vi "LithographyDriver.vi"(8 "error in (no error)":errorcluster) -> (0 "error out":errorcluster)   [LabVIEW 2016]
uses:
  Controls/lithography_Control.ctl
  litho folder/Global/Lithography Data.vi
  Desktop/Signal IO/SignalIO/tipvoltageglobal.vi
panel:
  in  "References":T1
  out "Current Object:":string
  out "Status:":string
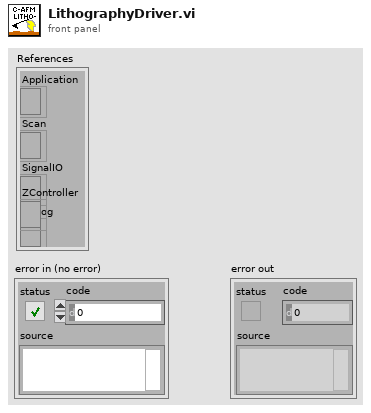
[diagram p1: front panel]
types:
  T1 = cluster{"Scan":refnum<k7>, "Lithog":refnum<k7>, "Application":refnum<k7>, "SignalIO":refnum<k7>, "ZController":refnum<k7>}
  T2 = typedef "lithography_Control.ctl" = enum16{"open_app", "create_ref", "current_pos", "init_litho", "get_init_pt", "clear_litho", "set_param", "move_tip", "create_queue", "clean_up_litho", "start_litho", "end"}
  T3 = cluster{"X_offset":dbl, "Y_offset":dbl, "init_x":dbl, "init_y":dbl, "voltage":dbl}
  T4 = cluster{"Name":string, "Litho":cluster{"X":dbl, "Y":dbl, "Speed":dbl, "Voltage":dbl}[]}[]
  T5 = cluster{"Lithography Data Out":cluster{"Name":string, "Litho":cluster{"X":dbl, "Y":dbl, "Speed":dbl, "Voltage":dbl}[]}[], "Values":cluster{"X_offset":dbl, "Y_offset":dbl, "init_x":dbl, "init_y":dbl, "voltage":dbl}, "References":cluster{"Scan":refnum<k7>, "Lithog":refnum<k7>, "Application":refnum<k7>, "SignalIO":refnum<k7>, "ZController":refnum<k7>}}
  T6 = cluster{"Pattern Data":cluster{"Name":string, "Litho":cluster{"X":dbl, "Y":dbl, "Speed":dbl, "Voltage":dbl}[]}, "Values":cluster{"X_offset":dbl, "Y_offset":dbl, "init_x":dbl, "init_y":dbl, "voltage":dbl}, "References":cluster{"Scan":refnum<k7>, "Lithog":refnum<k7>, "Application":refnum<k7>, "SignalIO":refnum<k7>, "ZController":refnum<k7>}}
  T7 = cluster{"X":dbl, "Y":dbl, "Speed":dbl, "Voltage":dbl}[]
  T8 = cluster{"X":dbl, "Y":dbl, "Speed":dbl, "Voltage":dbl}
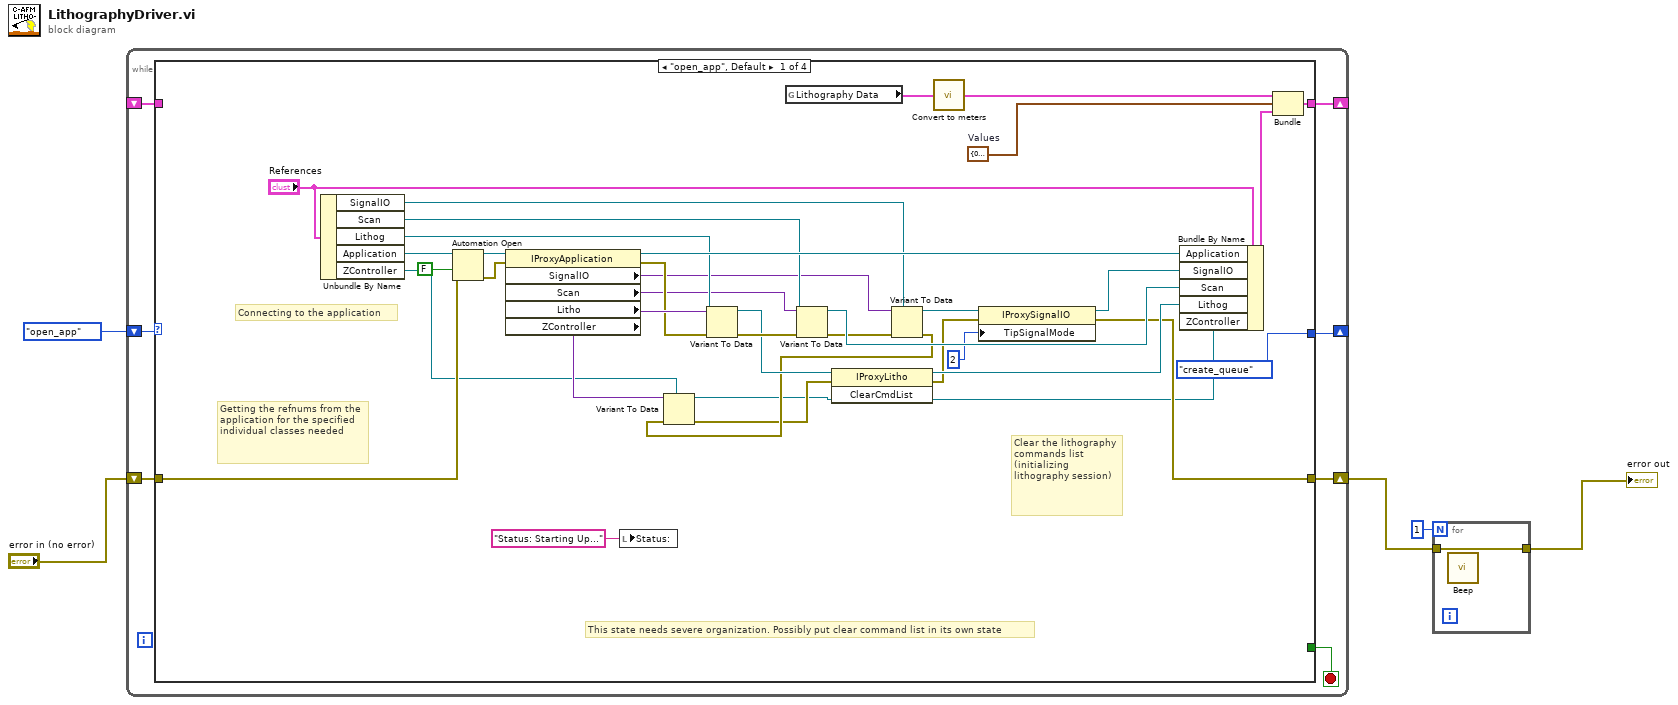
[diagram p0: block diagram]
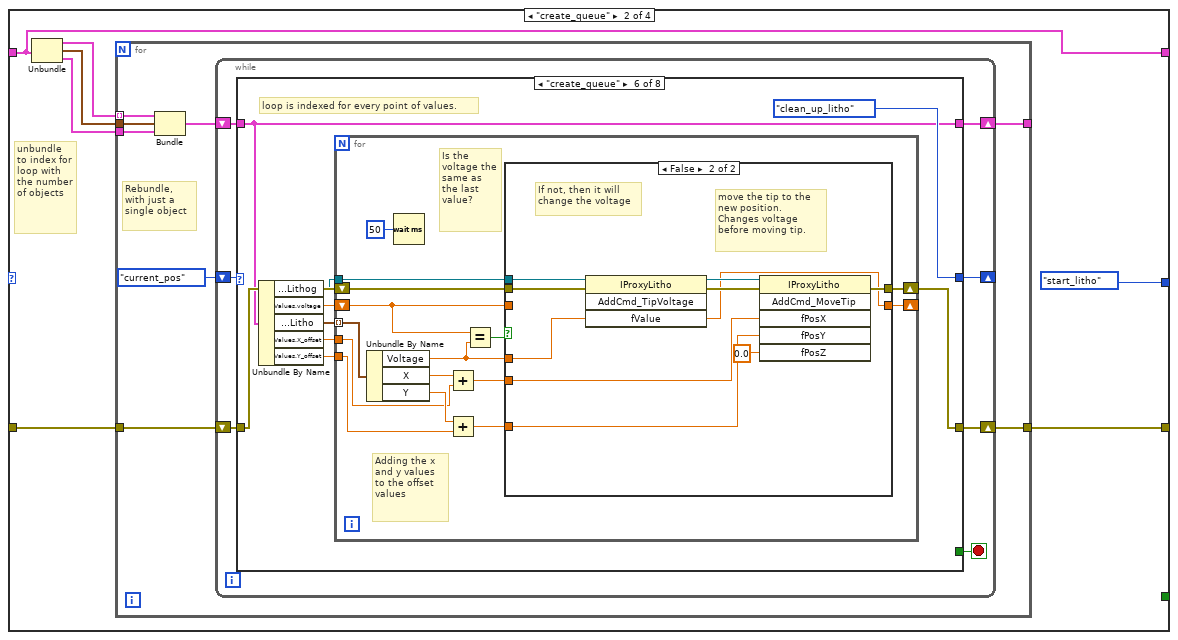
[diagram p2: hidden frame]
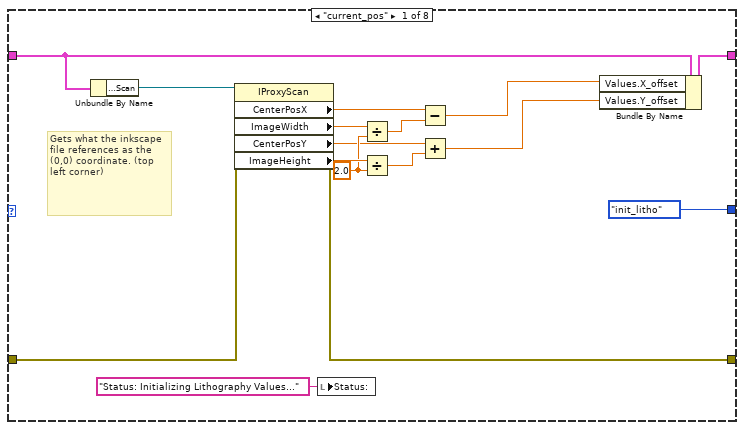
[diagram p3: hidden frame]
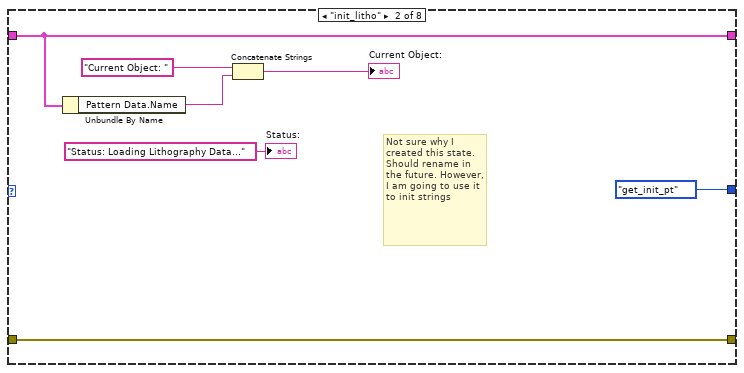
[diagram p4: hidden frame]
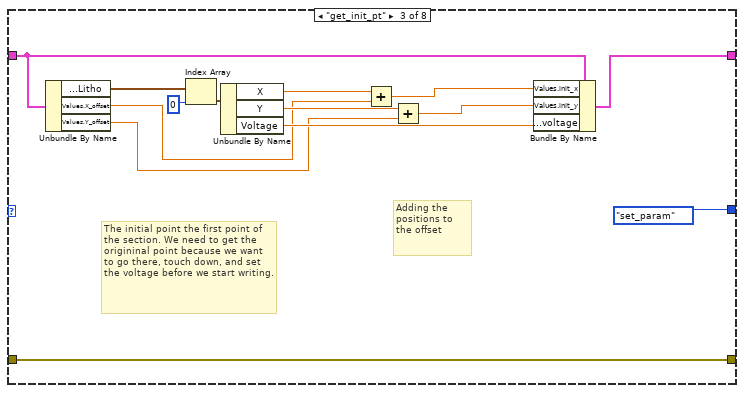
[diagram p5: hidden frame]
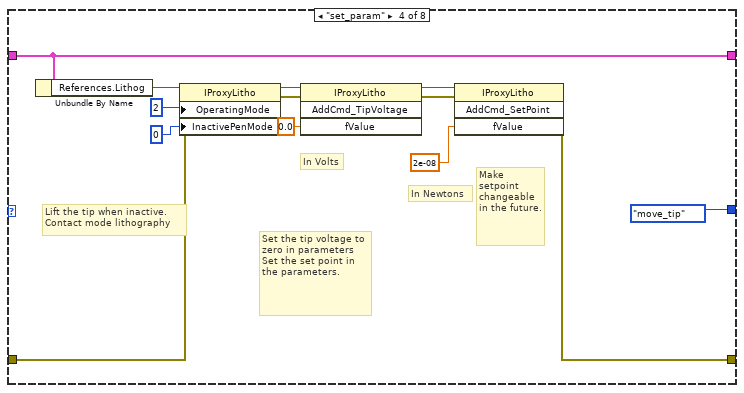
[diagram p6: hidden frame]
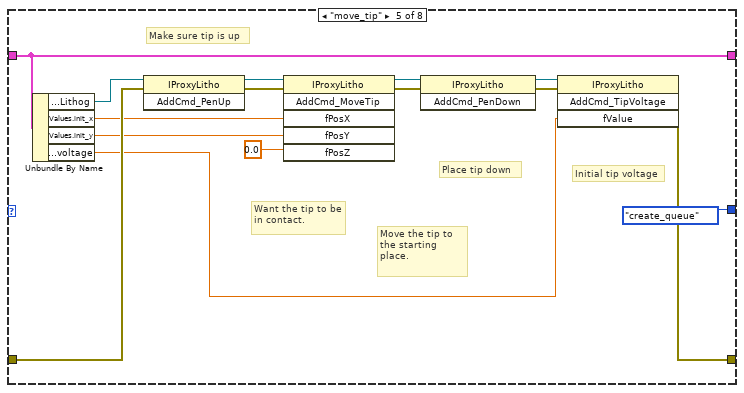
[diagram p7: hidden frame]
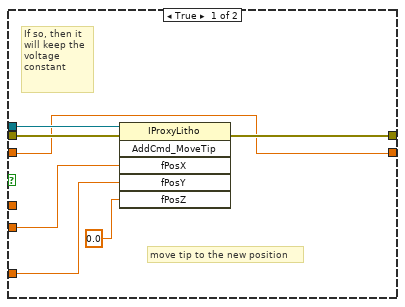
[diagram p8: hidden frame]
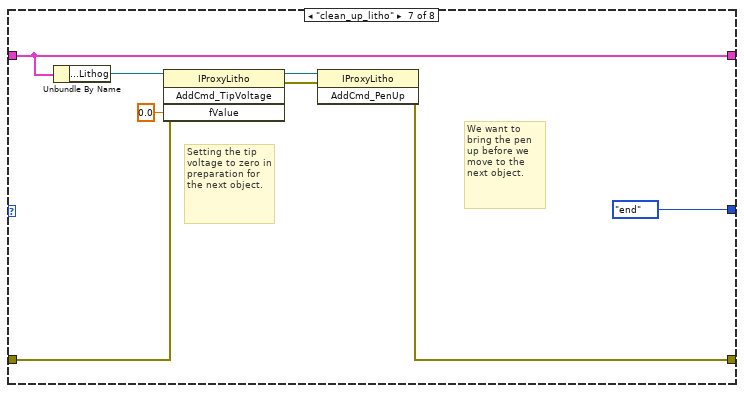
[diagram p9: hidden frame]
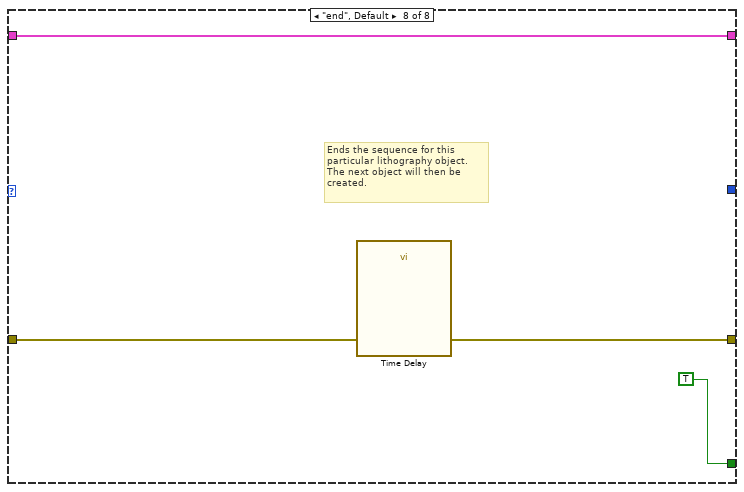
[diagram p10: hidden frame]
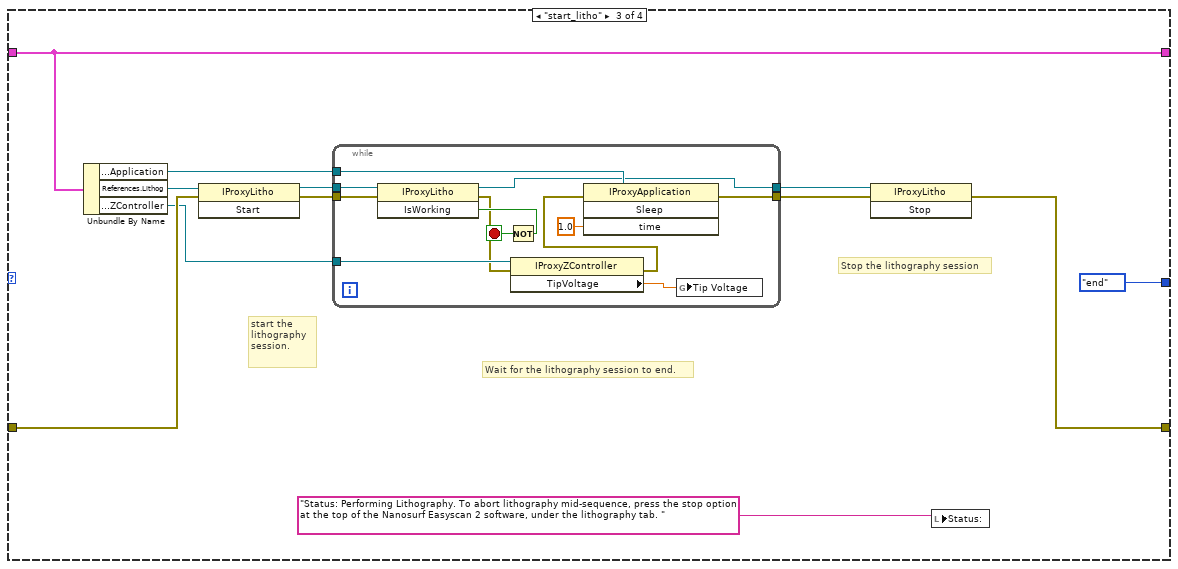
[diagram p11: hidden frame]
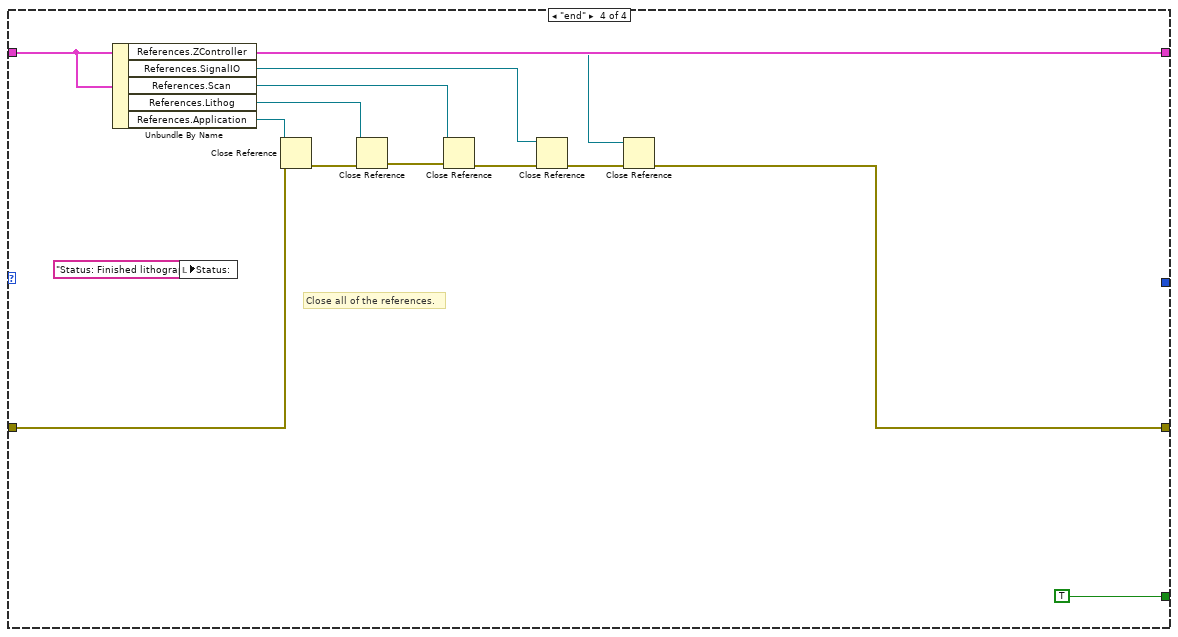
[diagram p12: hidden frame]
diagram:
  n1 = while {
    shift-right: [w7] -> _
    shift-left: lithography_Control."open_app" -> [w12]
    shift-right: [w10] -> w2
    shift-left: "error in (no error)" -> [w11]
    shift-right: [w9] -> _
    shift-left: _ -> [w8]
    stop <- w6 stop-if-true
    n2 = case shown="\"open_app\", Default" w12 {
      tunnel: w11 -> [w39 w55 w194 w220]
      tunnel: [w14 w54 w193 w213] -> w10
      tunnel: [w36 w49 w192 w222] -> w9
      tunnel: w8 -> [_ w49 w192 w222]
      tunnel: [lithography_Control."create_queue" lithography_Control."start_litho" lithography_Control."end" _] -> w7
      tunnel: [_ _ _ TRUE] -> w6
      frame "open_app", Default {
        w37 = T3 {"X_offset"=0.0, "Y_offset"=0.0, "init_x"=0.0, "init_y"=0.0, "voltage"=0.0}  # Values
        # "Getting the refnums from the application for the specified individual classes needed"
        # "Connecting to the application"
        # "Clear the lithography commands list\n(initializing lithography session)"
        # "This state needs severe organization. Possibly put clear command list in its own state"
        n3 = Unbundle By Name("References") -> ("SignalIO"=w26:refnum<k7>, "Scan"=w44:refnum<k7>, "Lithog"=w43:refnum<k7>, "Application"=w42:refnum<k7>, "ZController"=w17:refnum<k7>)
        n4 = Automation Open(error in (no error)=w39, Automation Refnum=w42, 9:FALSE ("open new instance (false)")) -> (Automation Refnum=w41:refnum<k7>, error out=w33:errorcluster)  [unwired: 1 in]
        n5 = property class="IProxyApplication"(reference=w41, error in=w33) -> (reference out=w45:refnum<k7>, error out=w32:errorcluster, "SignalIO"=w24:variant, "Scan"=w25:variant, "Litho"=w46:variant, "ZController"=w18:variant)
        n6 = local write "Status:"("Status: Starting Up..." ("Status")) -> ()
        n7 = Variant To Data(error in=w32, type=w43, Variant=w46) -> (data=w30:refnum<k7>, error out=w31:errorcluster)
        n8 = global read "Lithography Data.vi" "Lithography Data"() -> (w40:T4)
        n9 = Variant To Data(error in=w31, type=w44, Variant=w25) -> (data=w28:refnum<k7>, error out=w27:errorcluster)
        n10 = Variant To Data(error in=w27, type=w26, Variant=w24) -> (data=w22:refnum<k7>, error out=w16:errorcluster)
        n11 = Variant To Data(error in=w16, type=w17, Variant=w18) -> (data=w13:refnum<k7>, error out=w15:errorcluster)
        n12 = invoke class="IProxyLitho" method="ClearCmdList"(reference=w30, error in=w15) -> (reference out=w23:refnum<k7>, error out=w19:errorcluster)  [unwired: 1 in, 1 out]
        n13 = call "Convert to meters.vi"("Lithography Data In"=w40) -> ("Lithography Data Out"=w38:T4)
        n14 = property class="IProxySignalIO"(reference=w22, error in=w19, "TipSignalMode"=2) -> (reference out=w20:refnum<k7>, error out=w14:errorcluster)
        n15 = Bundle By Name(cluster="References", "Application"=w45, "SignalIO"=w20, "Scan"=w28, "Lithog"=w23, "ZController"=w13) -> (w35:T1)
        n16 = Bundle("Lithography Data Out"=w38, "Values"=w37, "References"=w35) -> (w36:T5)  [unwired: 1 in]
      }
      frame "create_queue" {
        # "unbundle to index for loop with the number of objects"
        n17 = Unbundle(w49) -> ("Lithography Data Out"=w53:T4, "Values"=w52:T3, "References"=w51:T1)
        n18 = for {
          tunnel: w55 -> [w62]
          tunnel: [w61] -> w54
          tunnel: [w60] -> _
          tunnel: w53 -> [w58] mode=indexing
          tunnel: w52 -> [w57]
          tunnel: w51 -> [w56]
          # "Rebundle, with just a single object"
          n19 = Bundle("Pattern Data"=w58, "Values"=w57, "References"=w56) -> (w59:T6)  [unwired: 1 in]
          n20 = while {
            shift-right: [w66] -> _
            shift-left: lithography_Control."current_pos" -> [w70]
            shift-right: [w68] -> w60
            shift-left: w59 -> [w69]
            shift-right: [w65] -> w61
            shift-left: w62 -> [w67]
            stop <- w64 stop-if-true
            n21 = case shown="\"create_queue\"" w70 {
              tunnel: w69 -> [w84 w91 w100 w119 w134 w141 w183 w188]
              tunnel: [w83 w91 w99 w119 w134 w141 w183 w188] -> w68
              tunnel: w67 -> [w82 w92 w106 w115 w128 w143 w178 w186]
              tunnel: [lithography_Control."init_litho" lithography_Control."get_init_pt" lithography_Control."set_param" lithography_Control."move_tip" lithography_Control."create_queue" lithography_Control."clean_up_litho" lithography_Control."end" _] -> w66
              tunnel: [w81 w92 w106 w109 w123 w142 w182 w187] -> w65
              tunnel: [_ _ _ _ _ _ _ TRUE] -> w64
              frame "current_pos" {
                w76 = 2.0 ("y")
                # "Gets what the inkscape file references as the (0,0) coordinate. (top left corner)"
                n22 = Unbundle By Name(w84) -> ("References.Scan"=w85:refnum<k7>)
                n23 = property class="IProxyScan"(reference=w85, error in=w82) -> (error out=w81:errorcluster, "CenterPosX"=w73:dbl, "ImageWidth"=w78:dbl, "CenterPosY"=w75:dbl, "ImageHeight"=w77:dbl)  [unwired: 1 out]
                n24 = local write "Status:"("Status: Initializing Lithography Values..." ("Status")) -> ()
                n25 = Divide(x=w78, y=w76) -> (x/y=w79:dbl)
                n26 = Divide(x=w77, y=w76) -> (x/y=w74:dbl)
                n27 = Subtract(x=w73, y=w79) -> (x-y=w72:dbl)
                n28 = Add(x=w75, y=w74) -> (x+y=w71:dbl)
                n29 = Bundle By Name(cluster=w84, "Values.X_offset"=w72, "Values.Y_offset"=w71) -> (w83:T6)
              }
              frame "init_litho" {
                # "Not sure why I created this state. Should rename in the future. However, I am going to use it to init strings"
                n30 = Unbundle By Name(w91) -> ("Pattern Data.Name"=w89:string)
                n31 = Concatenate Strings("Current Object: " ("string"), w89) -> (→"Current Object:":string)
                "Status:" <- "Status: Loading Lithography Data..." ("Status")
              }
              frame "get_init_pt" {
                # "Adding the positions to the offset"
                # "The initial point the first point of the section. We need to get the origininal point because we want to go there, touch down, and set the voltage before we start writing."
                n32 = Unbundle By Name(w100) -> ("Pattern Data.Litho"=w104:T7, "Values.X_offset"=w94:dbl, "Values.Y_offset"=w95:dbl)
                n33 = Index Array(array=w104, index=0) -> (element=w103:T8)
                n34 = Unbundle By Name(w103) -> ("X"=w102:dbl, "Y"=w101:dbl, "Voltage"=w96:dbl)
                n35 = Add(x=w102, y=w94) -> (x+y=w98:dbl)
                n36 = Add(x=w101, y=w95) -> (x+y=w97:dbl)
                n37 = Bundle By Name(cluster=w100, "Values.init_x"=w98, "Values.init_y"=w97, "Values.voltage"=w96) -> (w99:T6)
              }
              frame "set_param" {
                # "Make setpoint changeable in the future."
                # "In Volts"
                # "In Newtons"
                # "Set the tip voltage to zero in parameters\nSet the set point in the parameters."
                # "Lift the tip when inactive.\nContact mode lithography"
                n38 = Unbundle By Name(w119) -> ("References.Lithog"=w118:refnum<k7>)
                n39 = property class="IProxyLitho"(reference=w118, error in=w115, "OperatingMode"=2 ("InactivePenMode"), "InactivePenMode"=0 ("OperatingMode")) -> (reference out=w114:refnum<k7>, error out=w113:errorcluster)
                n40 = invoke class="IProxyLitho" method="AddCmd_TipVoltage"(reference=w114, error in=w113, "fValue"=0.0) -> (reference out=w111:refnum<k7>, error out=w110:errorcluster)  [unwired: 1 in, 2 out]
                n41 = invoke class="IProxyLitho" method="AddCmd_SetPoint"(reference=w111, error in=w110, "fValue"=2e-08 ("SetPoint")) -> (error out=w109:errorcluster)  [unwired: 1 in, 3 out]
              }
              frame "move_tip" {
                # "Initial tip voltage"
                # "Want the tip to be in contact."
                # "Make sure tip is up"
                # "Place tip down"
                # "Move the tip to the starting place."
                n42 = Unbundle By Name(w134) -> ("References.Lithog"=w127:refnum<k7>, "Values.init_x"=w126:dbl, "Values.init_y"=w125:dbl, "Values.voltage"=w121:dbl)
                n43 = invoke class="IProxyLitho" method="AddCmd_PenUp"(reference=w127, error in=w128) -> (reference out=w133:refnum<k7>, error out=w130:errorcluster)  [unwired: 1 in, 1 out]
                n44 = invoke class="IProxyLitho" method="AddCmd_MoveTip"(reference=w133, error in=w130, "fPosX"=w126, "fPosY"=w125, "fPosZ"=0.0) -> (reference out=w132:refnum<k7>, error out=w129:errorcluster)  [unwired: 1 in, 4 out]
                n45 = invoke class="IProxyLitho" method="AddCmd_PenDown"(reference=w132, error in=w129) -> (reference out=w124:refnum<k7>, error out=w122:errorcluster)  [unwired: 1 in, 1 out]
                n46 = invoke class="IProxyLitho" method="AddCmd_TipVoltage"(reference=w124, error in=w122, "fValue"=w121) -> (error out=w123:errorcluster)  [unwired: 1 in, 3 out]
              }
              frame "create_queue" {
                # "loop is indexed for every point of values."
                n47 = Unbundle By Name(w141) -> ("References.Lithog"=w139:refnum<k7>, "Values.voltage"=w138:dbl, "Pattern Data.Litho"=w136:T7, "Values.X_offset"=w140:dbl, "Values.Y_offset"=w137:dbl)
                n48 = for {
                  shift-right: [w157] -> w142
                  shift-left: w143 -> [w158]
                  tunnel: w139 -> [w159]
                  tunnel: w136 -> [w151] mode=indexing
                  tunnel: w140 -> [w146]
                  tunnel: w137 -> [w145]
                  shift-right: [w148] -> _
                  shift-left: w138 -> [w147]
                  # "Adding the x and y values to the offset values"
                  # "Is the voltage the same as the last value?"
                  n49 = Unbundle By Name(w151) -> ("Voltage"=w149:dbl, "X"=w156:dbl, "Y"=w154:dbl)
                  n50 = Wait (ms)(milliseconds to wait=u32 50) -> ()  [unwired: 1 out]
                  n51 = Add(x=w156, y=w146) -> (x+y=w155:dbl)
                  n52 = Add(x=w154, y=w145) -> (x+y=w153:dbl)
                  n53 = Equal?(x=w147, y=w149) -> (x = y?=w150:bool)
                  n54 = case shown="False" w150 {
                    tunnel: w159 -> [w166 w172]
                    tunnel: w158 -> [w165 w171]
                    tunnel: [w163 w175] -> w157
                    tunnel: w155 -> [w162 w174]
                    tunnel: w153 -> [w161 w173]
                    tunnel: w149 -> [_ w168]
                    tunnel: [w160 w167] -> w148
                    tunnel: w147 -> [w160 _]
                    frame True {
                      # "move tip to the new position"
                      # "If so, then it will keep the voltage constant"
                      n55 = invoke class="IProxyLitho" method="AddCmd_MoveTip"(reference=w166, error in=w165, "fPosX"=w162, "fPosY"=w161, "fPosZ"=0.0 ("fPosX")) -> (error out=w163:errorcluster)  [unwired: 1 in, 5 out]
                    }
                    frame False {
                      # "move the tip to the new position. Changes voltage before moving tip."
                      # "If not, then it will change the voltage"
                      n56 = invoke class="IProxyLitho" method="AddCmd_TipVoltage"(reference=w172, error in=w171, "fValue"=w168) -> (reference out=w169:refnum<k7>, error out=w170:errorcluster, "fValue"=w167:dbl)  [unwired: 1 in, 1 out]
                      n57 = invoke class="IProxyLitho" method="AddCmd_MoveTip"(reference=w169, error in=w170, "fPosX"=w174, "fPosY"=w173, "fPosZ"=0.0 ("fPosX")) -> (error out=w175:errorcluster)  [unwired: 1 in, 5 out]
                    }
                  }
                }
              }
              frame "clean_up_litho" {
                # "Setting the tip voltage to zero in preparation for the next object."
                # "We want to bring the pen up before we move to the next object."
                n58 = Unbundle By Name(w183) -> ("References.Lithog"=w181:refnum<k7>)
                n59 = invoke class="IProxyLitho" method="AddCmd_TipVoltage"(reference=w181, error in=w178, "fValue"=0.0) -> (reference out=w180:refnum<k7>, error out=w179:errorcluster)  [unwired: 1 in, 2 out]
                n60 = invoke class="IProxyLitho" method="AddCmd_PenUp"(reference=w180, error in=w179) -> (error out=w182:errorcluster)  [unwired: 1 in, 2 out]
              }
              frame "end", Default {
                # "Ends the sequence for this particular lithography object. The next object will then be created."
                n61 = call "Time Delay"("error in (no error)"=w186) -> ("error out"=w187:errorcluster)  [unwired: 10 in]
              }
            }
          }
        }
      }
      frame "start_litho" {
        # "Stop the lithography session"
        # "Wait for the lithography session to end."
        # "start the lithography session."
        n62 = Unbundle By Name(w192) -> ("References.Application"=w195:refnum<k7>, "References.Lithog"=w200:refnum<k7>, "References.ZController"=w189:refnum<k7>)
        n63 = invoke class="IProxyLitho" method="Start"(reference=w200, error in=w194) -> (reference out=w199:refnum<k7>, error out=w198:errorcluster)  [unwired: 1 in, 1 out]
        n64 = while {
          tunnel: w199 -> [w212]
          tunnel: [w205] -> w197
          tunnel: w198 -> [w210]
          tunnel: [w208] -> w196
          tunnel: w195 -> [w207]
          tunnel: w189 -> [w204]
          stop <- w209 stop-if-true
          n65 = invoke class="IProxyLitho" method="IsWorking"(reference=w212, error in=w210) -> (reference out=w205:refnum<k7>, error out=w203:errorcluster, "IsWorking"=w211:bool)  [unwired: 1 in]
          n66 = Not(x=w211) -> (.not. x?=w209:bool)
          n67 = property class="IProxyZController"(reference=w204, error in=w203) -> (error out=w202:errorcluster, "TipVoltage"=w201:dbl)  [unwired: 1 out]
          n68 = invoke class="IProxyApplication" method="Sleep"(reference=w207, error in=w202, "time"=1.0) -> (error out=w208:errorcluster)  [unwired: 1 in, 3 out]
          n69 = global write "tipvoltageglobal.vi" "Tip Voltage"(w201) -> ()
        }
        n70 = invoke class="IProxyLitho" method="Stop"(reference=w197, error in=w196) -> (error out=w193:errorcluster)  [unwired: 1 in, 2 out]
        n71 = local write "Status:"("Status: Performing Lithography. To abort lithography mid-sequence, press the stop option at the top of the Nanosurf Easyscan 2 software, under the lithography tab. " ("Status")) -> ()
      }
      frame "end" {
        # "Close all of the references."
        n72 = Unbundle By Name(w222) -> ("References.ZController"=w215:refnum<k7>, "References.SignalIO"=w216:refnum<k7>, "References.Scan"=w225:refnum<k7>, "References.Lithog"=w224:refnum<k7>, "References.Application"=w223:refnum<k7>)
        n73 = local write "Status:"("Status: Finished lithography.") -> ()
        n74 = Close Reference(reference=w223, error in (no error)=w220) -> (error out=w219:errorcluster)
        n75 = Close Reference(reference=w224, error in (no error)=w219) -> (error out=w226:errorcluster)
        n76 = Close Reference(reference=w225, error in (no error)=w226) -> (error out=w217:errorcluster)
        n77 = Close Reference(reference=w216, error in (no error)=w217) -> (error out=w214:errorcluster)
        n78 = Close Reference(reference=w215, error in (no error)=w214) -> (error out=w213:errorcluster)
      }
    }
  }
  n79 = for {
    N: 1 -> [_]
    tunnel: w2 -> [w227]
    tunnel: [w227] -> w1
    n80 = call <vilib>:"Beep.vi"() -> ()  [unwired: 12 in]
  }
  "error out" <- w1
